vi "sub_getIndexOfClickedElement.vi"(10 "NewVal":T1, 11 "OldVal":T1) -> (3 "index of clicked element":i32)   [LabVIEW 2018]
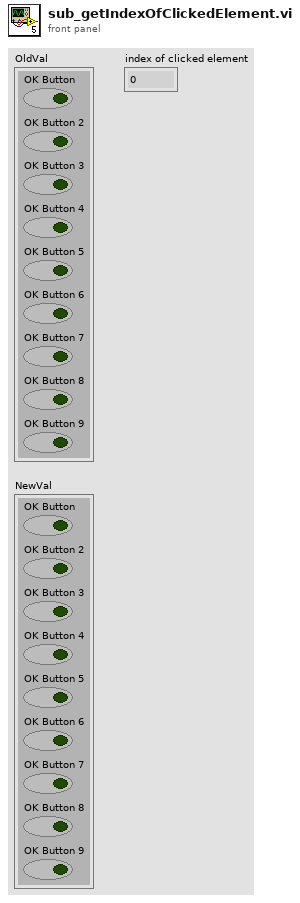
[diagram p1: front panel]
types:
  T1 = cluster{"OK Button":bool, "OK Button 2":bool, "OK Button 3":bool, "OK Button 4":bool, "OK Button 5":bool, "OK Button 6":bool, "OK Button 7":bool, "OK Button 8":bool, "OK Button 9":bool}
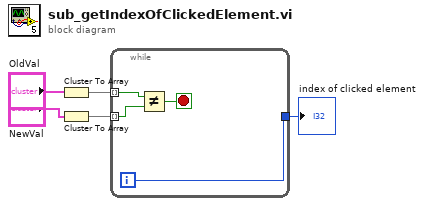
[diagram p0: block diagram]
diagram:
  n1 = Cluster To Array(cluster="OldVal") -> (array=w3:bool[])
  n2 = Cluster To Array(cluster="NewVal") -> (array=w4:bool[])
  n3 = while {
    tunnel: w3 -> [w8] mode=indexing
    tunnel: w4 -> [w9] mode=indexing
    tunnel: [w6] -> w5
    i -> [w6]
    stop <- w7 stop-if-true
    n4 = Not Equal?(x=w8, y=w9) -> (x != y?=w7:bool)
  }
  "index of clicked element" <- w5
